vi "Handle WebSocket Request.vi"(8 "error in (no error)":errorcluster, 10 "Request":refnum<class "Request.lvclass">, 11 "WebSocket Handler in":refnum<class "WebSocket Handler.lvclass">) -> (0 "error out":errorcluster, 1 "Response":refnum<class "Response.lvclass">, 2 "WebSocket":refnum<class "Websocket Server.lvclass">)   [LabVIEW 2020, in "HTTP Server.lvlib" / "WebSocket Handler.lvclass"]
uses:
  WebSocket Handler.lvclass
  lv-http-util/HTTP Utils/Request/Request.lvclass
  lv-http-util/HTTP Utils/Response/Response.lvclass
  lv-stream-websocket/Stream-Websocket/Websocket Server/Websocket Server.lvclass
  WebSocket Handler.lvclass/WebSocket Handler.ctl
  lv-stream-websocket/Stream-Websocket/WebSocketUpgradeResponse/WebSocketUpgradeResponse.lvclass
  C:/dev/lv20CE/relink/lv-http-util/HTTP Utils/Response/Response.lvclass
  lv-stream-websocket/Stream-Websocket/Stream-Websocket.lvlib
  lv-uri/URI/URI/URI.lvclass
  C:/dev/lv20CE/relink/lv-stream-websocket/Stream-Websocket/WebSocketUpgradeResponse/WebSocketUpgradeResponse.lvclass
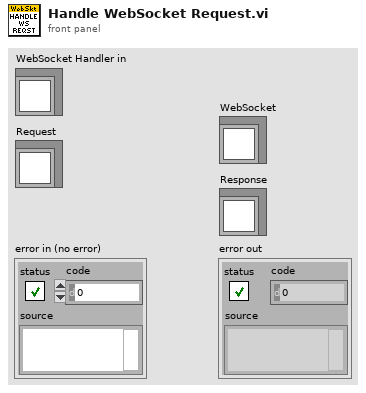
[diagram p1: front panel]
types:
  T1 = typedef "HTTP Server.lvlib/WebSocket Data.ctl" = cluster{"Buffered WS Map":map{string, refnum<class "Websocket Server.lvclass">}, "Message WS Map":map{string, refnum<class "Websocket Server.lvclass">}}
  T2 = map{string, refnum<class "Websocket Server.lvclass">}
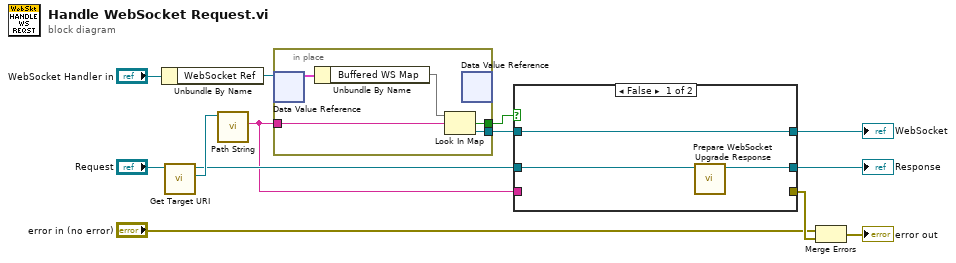
[diagram p0: block diagram]
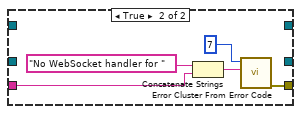
[diagram p2: hidden frame]
diagram:
  n1 = Unbundle By Name("WebSocket Handler in") -> ("WebSocket Ref"=w12:refnum<data-value>)
  n2 = call "Get Target URI.vi"("Request in"="Request") -> ("Target URI"=w10:refnum<class "URI.lvclass">, "Request out"=w7:refnum<class "Request.lvclass">)  [unwired: 8 in, 1 out]
  n3 = call "Path String.vi"("URI in"=w10) -> ("Path String"=w6:string)  [unwired: 9 in, 1 out]
  n4 = in-place {
    in-place-border: w6 -> [w16]
    in-place-border: [w15] -> w9
    in-place-border: [w14] -> w8
    n5 = in-place-dvr #1(w12) -> (w18:T1)  [unwired: 1 out]
    n6 = Unbundle By Name(w18) -> ("Buffered WS Map"=w17:T2)
    n7 = Look In Map(map=w17, key=w16) -> (key not found?=w15:bool, value=w14:refnum<class "Websocket Server.lvclass">)  [unwired: 1 in]
    n8 = in-place-dvr #1() -> ()  [unwired: 1 in, 2 out]
  }
  n9 = case shown="False" w9 {
    tunnel: w8 -> [w19 _]
    tunnel: w7 -> [w21 _]
    tunnel: w6 -> [_ w23]
    tunnel: [_ w22] -> w5
    tunnel: [w20 _] -> w2
    tunnel: [w19 _] -> w1
    frame False {
      n10 = call "Prepare WebSocket Upgrade Response.vi"("Request"=w21) -> ("WebSocket Response"=w20:refnum<class "WebSocketUpgradeResponse.lvclass">)  [unwired: 10 in]
    }
    frame True {
      n11 = Concatenate Strings("No WebSocket handler for " ("error message (\"\")"), w23) -> (w24:string)
      n12 = call <vilib>:"Error Cluster From Error Code.vi"("error message (\"\")"=w24, "error code (0)"=7) -> ("error out"=w22:errorcluster)  [unwired: 7 in]
    }
  }
  "Response" <- w2
  "WebSocket" <- w1
  n13 = Merge Errors("error in (no error)", w5) -> (→"error out":errorcluster)
